vi "Process Errors.vi"(8 "error in":errorcluster, 11 "RMXPowerSupply in":refnum<class "RMXPowerSupply.lvclass">) -> (0 "error out":errorcluster, 3 "RMXPowerSupply out":refnum<class "RMXPowerSupply.lvclass">)   [LabVIEW 2023]
uses:
  Support/Class/RMXPowerSupply.lvclass
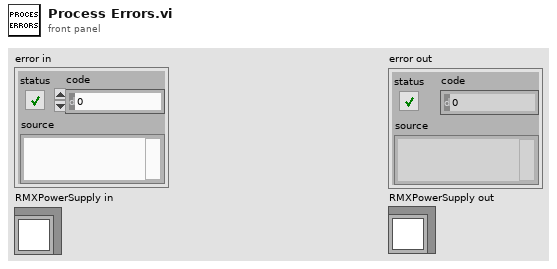
[diagram p1: front panel]
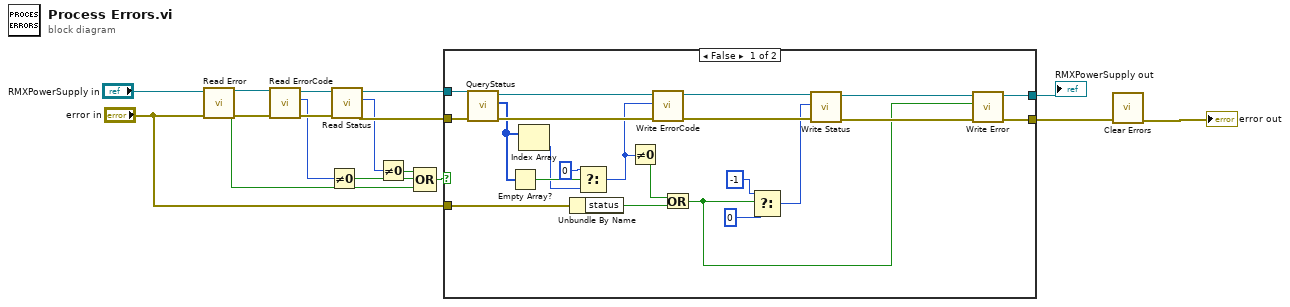
[diagram p0: block diagram]
diagram:
  n1 = call-dynamic "Read Error.vi"("error in (no error)"="error in", "RMXPowerSupply in"="RMXPowerSupply in") -> ("error out"=w14:errorcluster, "Error"=w6:bool, "RMXPowerSupply out"=w15:refnum<class "RMXPowerSupply.lvclass">)  [unwired: 7 in]
  n2 = call-dynamic "Read ErrorCode.vi"("error in (no error)"=w14, "RMXPowerSupply in"=w15) -> ("error out"=w9:errorcluster, "ErrorCode"=w5:i32, "RMXPowerSupply out"=w12:refnum<class "RMXPowerSupply.lvclass">)  [unwired: 7 in]
  n3 = Not Equal To 0?(x=w5) -> (x != 0?=w4:bool)
  n4 = call-dynamic "Read Status.vi"("error in (no error)"=w9, "RMXPowerSupply in"=w12) -> ("error out"=w10:errorcluster, "Status"=w7:i32, "RMXPowerSupply out"=w11:refnum<class "RMXPowerSupply.lvclass">)  [unwired: 7 in]
  n5 = Not Equal To 0?(x=w7) -> (x != 0?=w8:bool)
  n6 = Compound Arithmetic op=OR(w8, w4, w6) -> (w3:bool)
  n7 = case shown="False" w3 {
    tunnel: "error in" -> [w35 _]
    tunnel: [w28 w41] -> w13
    tunnel: [w27 w40] -> w2
    tunnel: w11 -> [w24 w40]
    tunnel: w10 -> [w23 w41]
    frame False {
      n8 = call-dynamic "QueryStatus.vi"("error in (no error)"=w23, "RMXPowerSupply in"=w24) -> ("error out"=w38:errorcluster, "Error Code"=w20:i32[], "RMXPowerSupply out"=w39:refnum<class "RMXPowerSupply.lvclass">)  [unwired: 6 in, 1 out]
      n9 = Empty Array?(array=w20) -> (empty?=w22:bool)
      n10 = Index Array(array=w20) -> (element=w19:i32)  [unwired: 1 in]
      n11 = Unbundle By Name(w35) -> ("status"=w34:bool)
      n12 = Select(t=0, s=w22, f=w19) -> (s? t:f=w18:i32)
      n13 = Not Equal To 0?(x=w18) -> (x != 0?=w33:bool)
      n14 = call-dynamic "Write ErrorCode.vi"("error in (no error)"=w38, "ErrorCode"=w18, "RMXPowerSupply in"=w39) -> ("error out"=w36:errorcluster, "RMXPowerSupply out"=w37:refnum<class "RMXPowerSupply.lvclass">)  [unwired: 7 in]
      n15 = Or(x=w33, y=w34) -> (x .or. y?=w25:bool)
      n16 = Select(t=-1 ("Status"), s=w25, f=0) -> (s? t:f=w30:i32)
      n17 = call-dynamic "Write Status.vi"("error in (no error)"=w36, "Status"=w30, "RMXPowerSupply in"=w37) -> ("error out"=w29:errorcluster, "RMXPowerSupply out"=w26:refnum<class "RMXPowerSupply.lvclass">)  [unwired: 7 in]
      n18 = call-dynamic "Write Error.vi"("error in (no error)"=w29, "Error"=w25, "RMXPowerSupply in"=w26) -> ("error out"=w28:errorcluster, "RMXPowerSupply out"=w27:refnum<class "RMXPowerSupply.lvclass">)  [unwired: 7 in]
    }
    frame True {
    }
  }
  "RMXPowerSupply out" <- w2
  n19 = call <vilib>:"Clear Errors.vi"("error in (no error)"=w13) -> ("error out"=→"error out":errorcluster)  [unwired: 5 in, 1 out]
